vi "niLvFpga_Download_NI 9149.vi"(0 "session in":u32, 11 "error in":errorcluster) -> (4 "session out":u32, 15 "error out":errorcluster)   [LabVIEW 2020]
uses:
  <vilib>/rvi/errors/niLvFpgaWhatHappensToTopLevelVI.ctl
  <vilib>/rvi/interface/common/niFpgaNodeNameForErrorReporting.ctl
  NiFpgaLv.dll
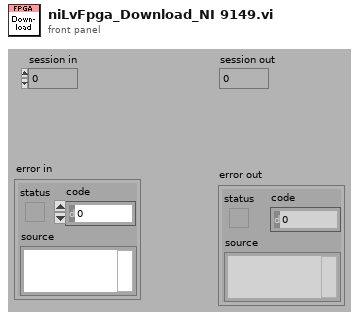
[diagram p1: front panel]
types:
  T1 = typedef "niLvFpgaWhatHappensToTopLevelVI.ctl" = enum16{"top level VI scripted behind XNode", "top level VI inlined behind XNode"}
  T2 = typedef "niFpgaNodeNameForErrorReporting.ctl" = enum16{"Open FPGA VI Reference", "Read/Write Control", "Invoke Method: Abort", "Invoke Method: Acknowledge IRQ", "Invoke Method: Download", "Invoke Method: FIFO.Configure", "Invoke Method: FIFO.Read", "Invoke Method: FIFO.Start", "Invoke Method: FIFO.Stop", "Invoke Method: FIFO.Write", "Invoke Method: Reset", "Invoke Method: Run", "Invoke Method: Wait on IRQ", "Close FPGA VI Reference", "Invoke Method: FIFO.Acquire Read Region", "Invoke Method: FIFO.Acquire Write Region"}
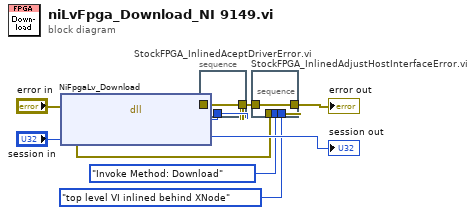
[diagram p0: block diagram]
diagram:
  n1 = dll-call lib="NiFpgaLv.*" fn="NiFpgaLv_Download" label="niLvFpgaDownload"(error in="error in", "sessionID"="session in") -> (error out=w7:errorcluster, "status"=w6:i32, "sessionID"=→"session out":u32)  [unwired: 2 in, 1 out]
  n2 = stacked-sequence "StockFPGA_InlinedAceptDriverError.vi" {
    tunnel: w7 -> [w10]
    tunnel: w6 -> [w12]
    tunnel: [w11] -> w5
    frame #0 {
      n3 = case shown="Default" w12 {
        selector: w12 -> [_ w14]
        tunnel: [w13 w16] -> w11
        tunnel: w10 -> [w13 w17]
        frame 0 {
        }
        frame Default {
          n4 = Greater Than 0?(x=w14) -> (x > 0?=w15:bool)
          n5 = call <vilib>:"Error Cluster From Error Code.vi"("is warning? (False)"=w15, "error in (no error)"=w17, "error code (0)"=w14) -> ("error out"=w16:errorcluster)  [unwired: 6 in]
        }
      }
    }
  }
  n6 = stacked-sequence "StockFPGA_InlinedAdjustHostInterfaceError.vi" {
    tunnel: w5 -> [w23]
    tunnel: "error in" -> [w20]
    tunnel: niFpgaNodeNameForErrorReporting."Invoke Method: Download" ("node name for error reporting") -> [w18]
    tunnel: niLvFpgaWhatHappensToTopLevelVI."top level VI inlined behind XNode" ("what happens to top level VI") -> [w19]
    tunnel: [w21] -> w1
    frame #0 {
      n7 = Unbundle By Name(w23) -> ("code"=w22:i32)
      n8 = case shown="Default" w22 {
        tunnel: [w24 w29] -> w21
        tunnel: w20 -> [w24 w28]
        tunnel: w19 -> [_ w27]
        tunnel: w18 -> [_ w26]
        tunnel: w23 -> [_ w25]
        frame 0 {
        }
        frame Default {
          n9 = call <vilib>:"niLvFpgaAdjustHostInterfaceError.vi"("error in"=w25, "prior error in"=w28, "node name for error reporting"=w26, "what happens to top level VI"=w27) -> ("error out"=w29:errorcluster)  [unwired: 11 in]
        }
      }
    }
  }
  "error out" <- w1
